vi "set_fiber_spiral_parameters.vi"(8 "error in (no error)":errorcluster, 10 "Fiber spiral parameters":T1={"Fiber Frequency"=2200, "Imaging Periods"=100, "Settling Periods"=50, "Resting Periods"=30, "Amplitude X"=0.5, "Amplitude Y"=0.5, "Phase difference"=90.0, "Initial Amplitude X"=0.0, "Initial Amplitude Y"=0.0} {"Initial Amplitude Y" min=0.0 max=3.0 step=0.1; "Initial Amplitude X" min=0.0 max=3.0 step=0.1; "Phase difference" min=0.0 max=360.0 step=5.0; "Amplitude Y" min=0.0 max=3.0 step=0.1; "Amplitude X" min=0.0 max=3.0 step=0.1}, 11 "FPGAWrapperRK120511Fiber_Spiral in":refnum<class "FPGAWrapperRK110512Fiber_Spiral.lvclass">) -> (0 "error out":errorcluster, 3 "FPGAWrapperRK120511Fiber_Spiral out":refnum<class "FPGAWrapperRK110512Fiber_Spiral.lvclass">)   [LabVIEW 2010, in "FPGAWrapperRK110512Fiber_Spiral.lvclass"]
uses:
  FPGAWrapperRK110512Fiber_Spiral.lvclass
  fiber_spiral_parameters.ctl
  <vilib>/rvi/interface/nirviReadWriteControl/nirviReadWriteControl.xnode
  FPGA_VI_Reference.ctl
  <vilib>/rvi/interface/common/niFpgaNodeNameForErrorReporting.ctl
  <vilib>/rvi/errors/niLvFpgaWhatHappensToTopLevelVI.ctl
  <vilib>/Utility/error.llb/Error Cluster From Error Code.vi
  <vilib>/rvi/errors/niLvFpgaAdjustHostInterfaceError.vi
  NiFpgaLv.dll
panel:
  # "[Hz]"
  # "[V]"
  # "[V]"
  # "[deg]"
  # "[V]"
  # "[V]"
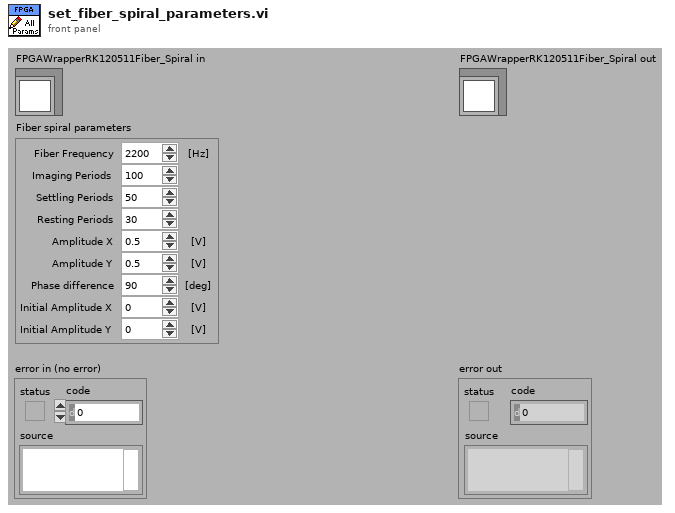
[diagram p1: front panel]
types:
  T1 = typedef "FPGAWrapperRK110512Fiber_Spiral.lvclass/fiber_spiral_parameters.ctl" = cluster{"Fiber Frequency":u16, "Imaging Periods":u16, "Settling Periods":u16, "Resting Periods":u16, "Amplitude X":dbl, "Amplitude Y":dbl, "Phase difference":dbl, "Initial Amplitude X":dbl, "Initial Amplitude Y":dbl}
  T2 = typedef "niFpgaNodeNameForErrorReporting.ctl" = enum16{"Open FPGA VI Reference", "Read/Write Control", "Invoke Method: Abort", "Invoke Method: Acknowledge IRQ", "Invoke Method: Download", "Invoke Method: FIFO.Configure", "Invoke Method: FIFO.Read", "Invoke Method: FIFO.Start", "Invoke Method: FIFO.Stop", "Invoke Method: FIFO.Write", "Invoke Method: Reset", "Invoke Method: Run", "Invoke Method: Wait on IRQ", "Close FPGA VI Reference"}
  T3 = typedef "niLvFpgaWhatHappensToTopLevelVI.ctl" = enum16{"top level VI scripted behind XNode", "top level VI inlined behind XNode"}
  T4 = typedef "FPGA Cycle Parameters XY.ctl" = cluster{"FPGA Cycle Parameters X":T5, "FPGA Cycle Parameters Y":T5}
  T5 = typedef "FPGA Cycle Parameters.ctl" = cluster{"Imaging cycles":i32, "Settling cycles":i32, "Resting cycles":i32, "Phase advance per cycle":fxp<+,32,0>, "Imaging Multiplier advance per cycle":fxp<+/-,32,0>, "Settling Multiplier advance per cycle":fxp<+/-,32,0>, "Imaging Initial Multiplier":fxp<+/-,43,12>, "Initial Phase":fxp<+,32,1>}
  T6 = typedef "FPGAWrapperRK110512Fiber_Spiral.lvclass/FPGA_VI_Reference.ctl" = refnum<k20>
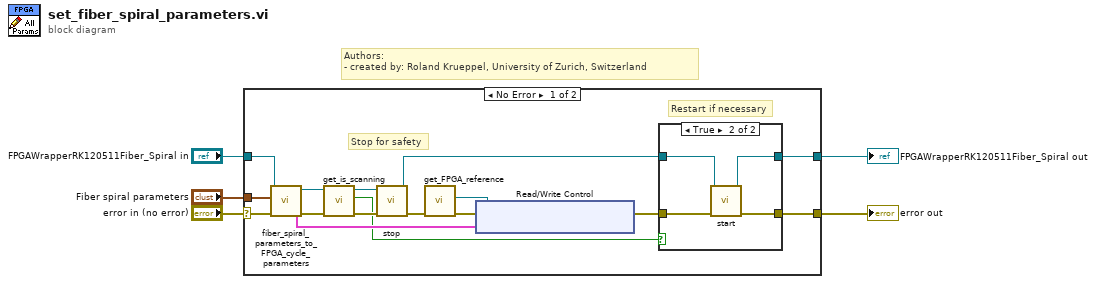
[diagram p0: block diagram]
diagram:
  # "Authors: \n- created by: Roland Krueppel, University of Zurich, Switzerland"
  n1 = case shown="No Error" "error in (no error)" {
    selector: "error in (no error)" -> [w21 w72]
    tunnel: [w6 w73] -> w3
    tunnel: "FPGAWrapperRK120511Fiber_Spiral in" -> [w19 w73]
    tunnel: "Fiber spiral parameters" -> [w20 _]
    tunnel: [w8 w72] -> w1
    frame No Error {
      # "Restart if necessary"
      # "Stop for safety"
      n2 = call-dynamic "fiber_spiral_parameters_to_FPGA_cycle_parameters.vi"("error in (no error)"=w21, "Fiber spiral parameters"=w20, "FPGAWrapperRK120511Fiber_Spiral in"=w19) -> ("error out"=w14:errorcluster, "FPGA Cycle Parameters XY"=w16:T4, "FPGAWrapperRK120511Fiber_Spiral out"=w13:refnum<class "FPGAWrapperRK110512Fiber_Spiral.lvclass">)  [unwired: 6 in]
      n3 = call-dynamic "get_is_scanning.vi"("error in (no error)"=w14, "FPGAWrapperRK110512Fiber_Spiral in"=w13) -> ("error out"=w12:errorcluster, "Scanning?"=w10:bool, "FPGAWrapperRK110512Fiber_Spiral out"=w11:refnum<class "FPGAWrapperRK110512Fiber_Spiral.lvclass">)  [unwired: 7 in]
      n4 = call-dynamic "stop.vi"("error in (no error)"=w12, "FPGAWrapperRK120511Fiber_Spiral in"=w11) -> ("error out"=w15:errorcluster, "FPGAWrapperRK120511Fiber_Spiral out"=w7:refnum<class "FPGAWrapperRK110512Fiber_Spiral.lvclass">)  [unwired: 8 in]
      n5 = call "get_FPGA_reference.vi"("error in (no error)"=w15) -> ("error out"=w17:errorcluster, "FPGA VI Reference"=w18:T6)  [unwired: 8 in, 1 out]
      n6 = xnode "Read/Write Control"("FPGA VI Reference In"=w18, "error in"=w17, "FPGA Cycle Parameters XY"=w16) -> ("error out"=w9:errorcluster)  [unwired: 1 out]
      n7 = case shown="True" w10 {
        tunnel: w9 -> [w22 w27]
        tunnel: [w22 w26] -> w8
        tunnel: w7 -> [w23 w25]
        tunnel: [w23 w24] -> w6
        frame False {
        }
        frame True {
          n8 = call-dynamic "start.vi"("error in (no error)"=w27, "FPGAWrapperRK120511Fiber_Spiral in"=w25) -> ("error out"=w26:errorcluster, "FPGAWrapperRK120511Fiber_Spiral out"=w24:refnum<class "FPGAWrapperRK110512Fiber_Spiral.lvclass">)  [unwired: 8 in]
        }
      }
    }
    frame Error {
    }
  }
  "error out" <- w1
  "FPGAWrapperRK120511Fiber_Spiral out" <- w3
